vi "Read ShortTestResult.vi"(8 "error in (no error)":errorcluster, 11 "TestReport in":refnum<class "TestReport.lvclass">) -> (0 "error out":errorcluster, 2 "ShortTestReport":string[](array[string]), 3 "TestReport out":refnum<class "TestReport.lvclass">)   [LabVIEW 2019, in "LocalReport.lvlib" / "TestReport.lvclass"]
uses:
  TestReport.lvclass
  TestReport.lvclass/TestReport.ctl
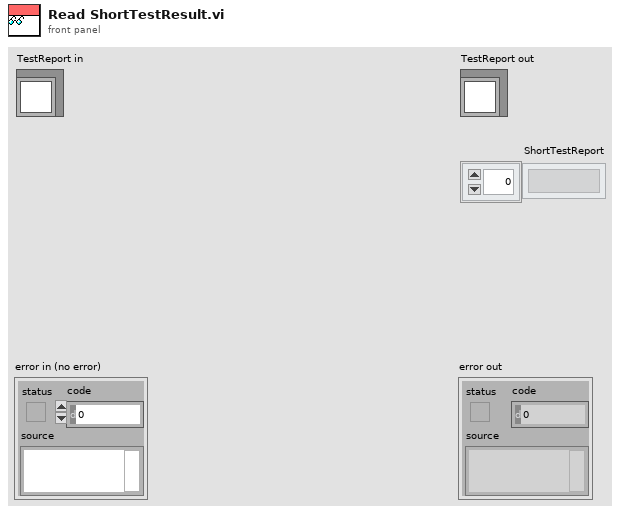
[diagram p1: front panel]
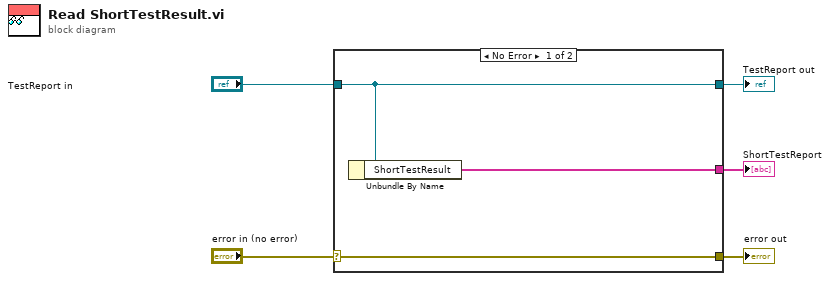
[diagram p0: block diagram]
diagram:
  n1 = case shown="No Error" "error in (no error)" {
    selector: "error in (no error)" -> [w8 w9]
    tunnel: [w8 w9] -> w4
    tunnel: [w7 w10] -> w2
    tunnel: "TestReport in" -> [w7 w10]
    tunnel: [w6 _] -> w1
    frame No Error {
      n2 = Unbundle By Name(w7) -> ("ShortTestResult"=w6:string[])
    }
    frame Error {
    }
  }
  "error out" <- w4
  "TestReport out" <- w2
  "ShortTestReport" <- w1
